vi "Config XML.vi"(1 "from file":T1 {"payload" format="%02x"}, 7 "Program":string, 8 "error in (no error)":errorcluster caption="错误输入（无错误）", 9 "NAD":u8 format="%.0x", 10 "Send Data":refnum<vi>, 11 "XML File Path":path caption="XML文件路径") -> (3 "XML File Path(duplicate)":path caption="XML文件路径（副本）")   [LabVIEW 2018]
uses:
  Crl/LIN_DataType.ctl
  <vilib>/Utility/xml.llb/Read From XML File(string).vi
  <vilib>/Utility/xml.llb/Write to XML File(string).vi
panel:
  in  "NAD":u8 format="%.0x"
  in  "exit":bool
  in  "Inset":bool
  in  "current":T1 {"payload" format="%02x"}
  # "ms"
  # "ms"
  # "ms"
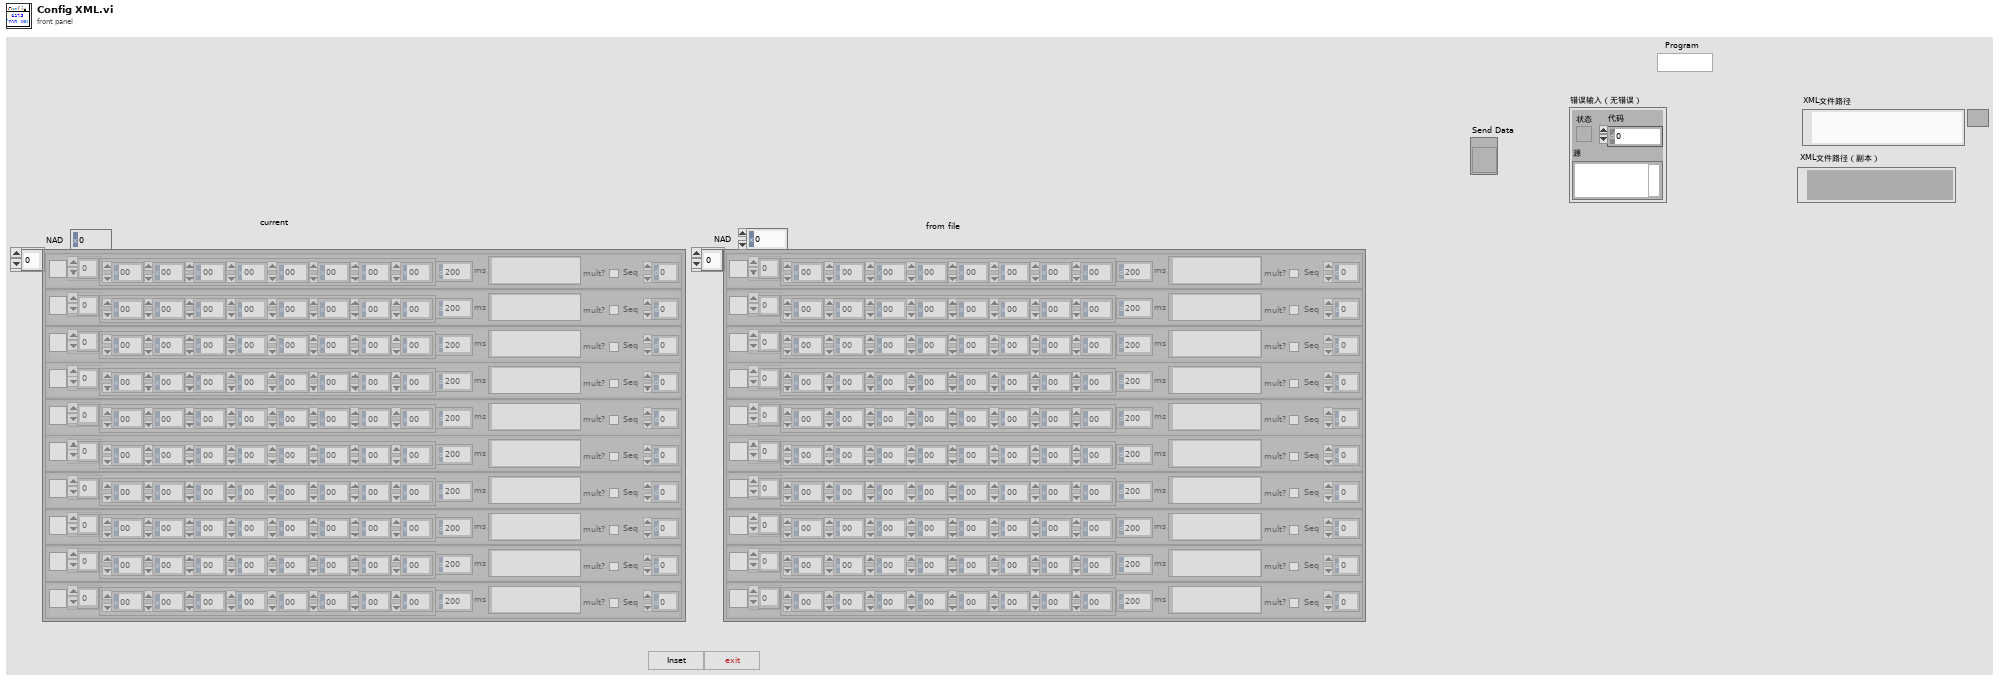
[diagram p1: front panel]
types:
  T1 = typedef "LIN_DataType.ctl" = cluster{"send?":bool, "payload":u8[], "Delays":u32, "Note":string, "mult?":bool, "Seq":i32}[]
  T2 = cluster{"current":refnum<vi>, "from file":refnum<vi>, "XML File Path(duplicate)":path, "error out":errorcluster, "NAD":u8}
  T3 = cluster{"send?":bool, "payload":u8[], "Delays":u32, "Note":string, "mult?":bool, "Seq":i32}
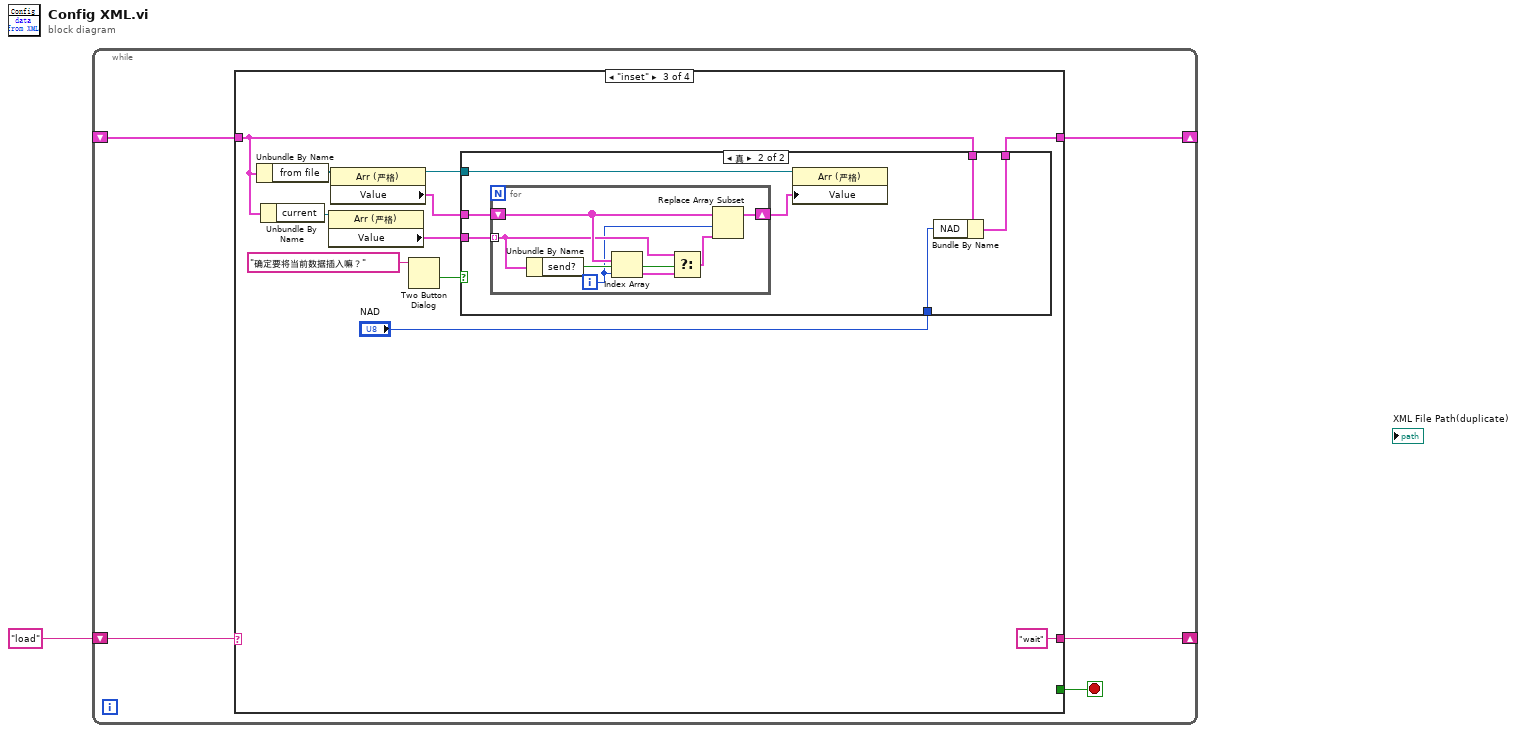
[diagram p0: block diagram]
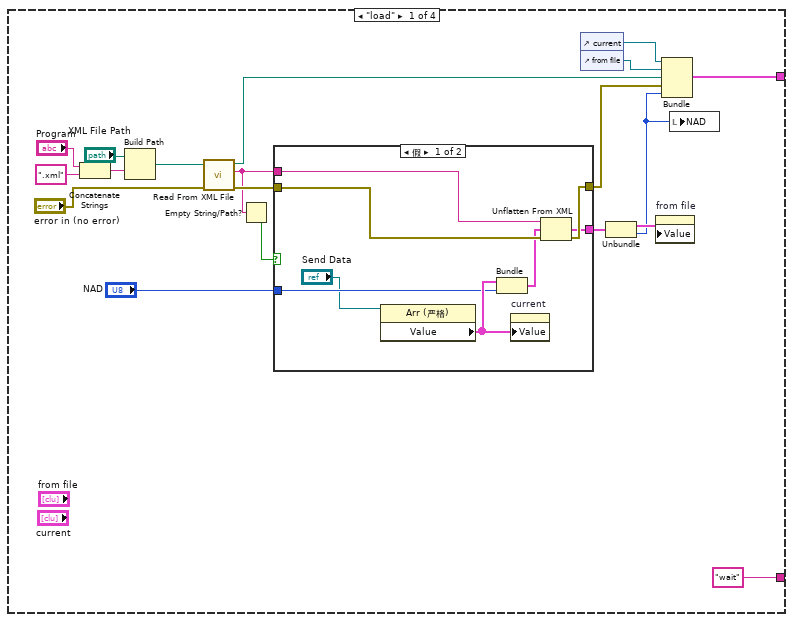
[diagram p2: hidden frame]
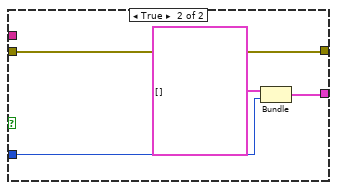
[diagram p3: hidden frame]
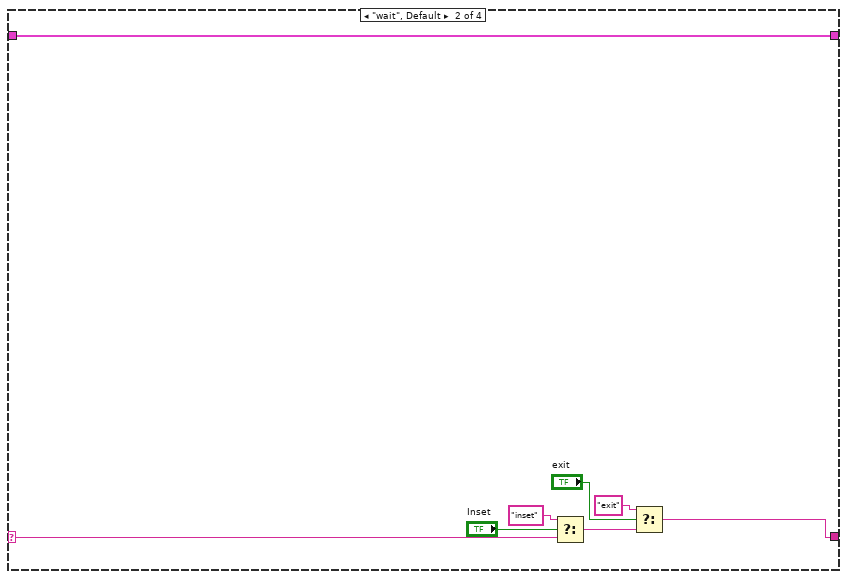
[diagram p4: hidden frame]
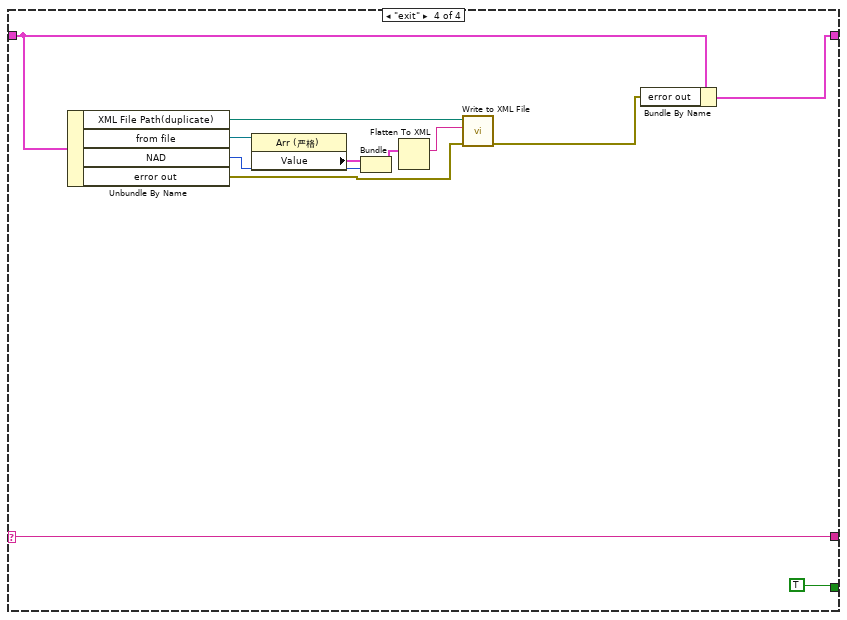
[diagram p6: hidden frame]
diagram:
  n1 = while {
    shift-right: [w5] -> _
    shift-left: "load" -> [w6]
    shift-right: [w4] -> _
    shift-left: _ -> [w3]
    stop <- w2 stop-if-true
    n2 = case shown="\"inset\"" w6 {
      selector: w6 -> [_ w40 _ w83]
      tunnel: ["wait" w39 "wait" w83] -> w5
      tunnel: [w21 w38 w47 w77] -> w4
      tunnel: w3 -> [_ w38 w48 w78]
      tunnel: [_ _ _ TRUE] -> w2
      frame "load" {
        n3 = Concatenate Strings("Program", ".xml" ("字符串")) -> (w15:string)
        n4 = Build Path(base path="XML File Path", name or relative path=w15) -> (appended path=w11:path)
        n5 = call-poly <vilib>:"Read From XML File.vi"("error in (no error)"="error in (no error)", "XML File Path"=w11) -> ("error out"=w25:errorcluster, "XML Elements"=w10:string, "XML File Path(duplicate)"=w22:path)  [unwired: 7 in]
        n6 = Empty String/Path?(string/path=w10) -> (empty?=w9:bool)
        n7 = case shown="假" w9 {
          tunnel: w25 -> [w33 w37]
          tunnel: [w32 w37] -> w14
          tunnel: [w29 w35] -> w13
          tunnel: w10 -> [w28 _]
          tunnel: "NAD" -> [w27 w36]
          frame False {
            n8 = property class="Arr (严格)"(reference="Send Data") -> ("Value"=w31:T1)  [unwired: 1 in, 2 out]
            n9 = Bundle("Value"=w31, "NAD"=w27) -> (w30:cluster{"Value":T1, "NAD":u8})  [unwired: 1 in]
            n10 = property on="current" class="Arr (严格)"("Value"=w31) -> ()  [unwired: 2 in, 2 out]
            n11 = Unflatten From XML(xml string=w28, type=w30, error in (no error)=w33) -> (value=w29:cluster{"Value":T1, "NAD":u8}, error out=w32:errorcluster)
          }
          frame True {
            n12 = Bundle("值"=T1 [], "NAD"=w36) -> (w35:cluster{"值":T1, "NAD":u8})  [unwired: 1 in]
          }
        }
        n13 = control-ref of="current"() -> (w20:refnum<vi>)
        n14 = control-ref of="from file"() -> (w19:refnum<vi>)
        n15 = Unbundle(w13) -> ("值"=w12:T1, "NAD"=w7:u8)
        n16 = property on="from file" class="Arr (严格)"("Value"=w12) -> ()  [unwired: 2 in, 2 out]
        n17 = Bundle("current"=w20, "from file"=w19, "XML File Path(duplicate)"=w22, "error out"=w14, "NAD"=w7) -> (w21:T2)  [unwired: 1 in]
        n18 = local write "NAD"(w7) -> ()
      }
      frame "wait", Default {
        n19 = Select(t="inset", s="Inset", f=w40) -> (s? t:f=w42:string)
        n20 = Select(t="exit", s="exit", f=w42) -> (s? t:f=w39:string)
      }
      frame "inset" {
        n21 = Unbundle By Name(w48) -> ("from file"=w54:refnum<vi>)
        n22 = Unbundle By Name(w48) -> ("current"=w56:refnum<vi>)
        n23 = property class="Arr (严格)"(reference=w56) -> ("Value"=w55:T1)  [unwired: 1 in, 2 out]
        n24 = property class="Arr (严格)"(reference=w54) -> (reference out=w52:refnum<vi>, "Value"=w53:T1)  [unwired: 1 in, 1 out]
        n25 = Two Button Dialog(message="确定要将当前数据插入嘛？" ("消息")) -> (T button?=w50:bool)  [unwired: 2 in]
        n26 = case shown="真" w50 {
          tunnel: w55 -> [_ w64]
          tunnel: w53 -> [_ w63]
          tunnel: w52 -> [_ w62]
          tunnel: w48 -> [w57 w60]
          tunnel: [w57 w59] -> w47
          tunnel: "NAD" -> [_ w58]
          frame False {
          }
          frame True {
            n27 = for {
              tunnel: w64 -> [w69] mode=indexing
              shift-right: [w65] -> w61
              shift-left: w63 -> [w71]
              i -> [w66]
              n28 = Unbundle By Name(w69) -> ("send?"=w70:bool)
              n29 = Index Array(array=w71, index=w66) -> (element=w68:T3)
              n30 = Select(t=w69, s=w70, f=w68) -> (s? t:f=w67:T3)
              n31 = Replace Array Subset(array=w71, new element=w67, index=w66) -> (w65:T1)
            }
            n32 = property class="Arr (严格)"(reference=w62, "Value"=w61) -> ()  [unwired: 1 in, 2 out]
            n33 = Bundle By Name(cluster=w60, "NAD"=w58) -> (w59:T2)
          }
        }
      }
      frame "exit" {
        n34 = Unbundle By Name(w78) -> ("XML File Path(duplicate)"=w80:path, "from file"=w81:refnum<vi>, "NAD"=w74:u8, "error out"=w72:errorcluster)
        n35 = property class="Arr (严格)"(reference=w81) -> ("Value"=w75:T1)  [unwired: 1 in, 2 out]
        n36 = Bundle("Value"=w75, "NAD"=w74) -> (w73:cluster{"Value":T1, "NAD":u8})  [unwired: 1 in]
        n37 = Flatten To XML(anything=w73) -> (xml string=w79:string)
        n38 = call-poly <vilib>:"Write to XML File.vi"("error in (no error)"=w72, "XML Input"=w79, "XML File Path"=w80) -> ("error out"=w76:errorcluster)  [unwired: 6 in, 2 out]
        n39 = Bundle By Name(cluster=w78, "error out"=w76) -> (w77:T2)
      }
    }
  }
